vi "Ball-Goal Impact Penalty.vi"(9 "Field Length":dbl, 10 "Ball":T1, 11 "Ball Velocity":dbl[](array[numeric])) -> (3 "Y Collision":dbl)   [LabVIEW 2016]
uses:
  Core/AI Ball.ctl
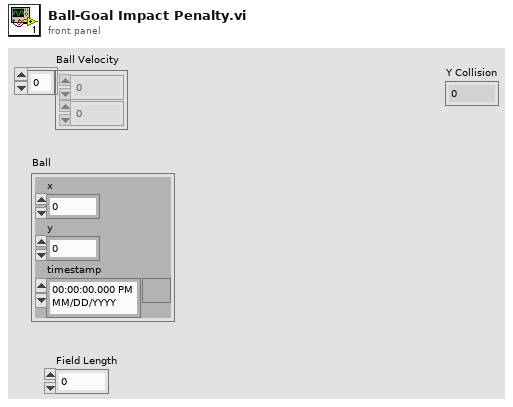
[diagram p1: front panel]
types:
  T1 = typedef "AI Ball.ctl" = cluster{"x":dbl, "y":dbl, "timestamp":timestamp}
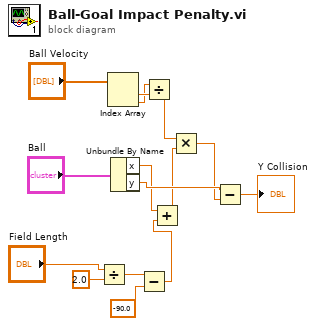
[diagram p0: block diagram]
diagram:
  n1 = Divide(x="Field Length", y=2.0) -> (x/y=w3:dbl)
  n2 = Index Array(array="Ball Velocity") -> (element #1=w12:dbl, element #2=w11:dbl)  [unwired: 2 in]
  n3 = Unbundle By Name("Ball") -> ("x"=w7:dbl, "y"=w13:dbl)
  n4 = Subtract(x=w3, y=-90.0) -> (x-y=w1:dbl)
  n5 = Divide(x=w11, y=w12) -> (x/y=w10:dbl)
  n6 = Add(x=w7, y=w1) -> (x+y=w6:dbl)
  n7 = Multiply(x=w10, y=w6) -> (x*y=w9:dbl)
  n8 = Subtract(x=w13, y=w9) -> (x-y=→"Y Collision":dbl)
